vi "Get Data_To_Encrypt.vi"(8 "error in (no error)":errorcluster caption="entrée d'erreur (pas d'erreur)", 11 "Cryptographic Hash (Default) en entrée":refnum<class "Cryptographic Hash (Default).lvclass">) -> (0 "error out":errorcluster caption="sortie d'erreur", 2 "Data_To_Encrypt":string, 3 "Cryptographic Hash (Default) en sortie":refnum<class "Cryptographic Hash (Default).lvclass">)   [LabVIEW 2020, in "Library Cryptographic Hash.lvlib" / "Cryptographic Hash (Default).lvclass"]
uses:
  Cryptographic Hash (Default).lvclass
  Cryptographic Hash (Default).lvclass/Cryptographic Hash (Default).ctl
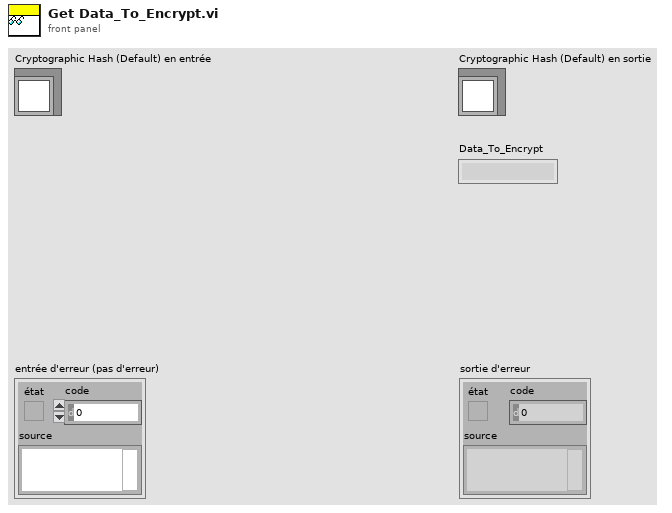
[diagram p1: front panel]
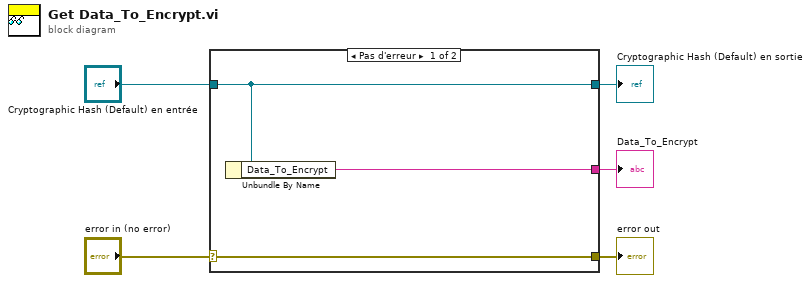
[diagram p0: block diagram]
diagram:
  n1 = case shown="Pas d'erreur" "error in (no error)" {
    selector: "error in (no error)" -> [w8 w9]
    tunnel: [w8 w9] -> w4
    tunnel: [w7 w10] -> w2
    tunnel: "Cryptographic Hash (Default) en entrée" -> [w7 w10]
    tunnel: [w6 _] -> w1
    frame No Error {
      n2 = Unbundle By Name(w7) -> ("Data_To_Encrypt"=w6:string)
    }
    frame Error {
    }
  }
  "error out" <- w4
  "Cryptographic Hash (Default) en sortie" <- w2
  "Data_To_Encrypt" <- w1
